vi "CSM - List Log Filter Rules As Strings.vi"(8 "Error in":errorcluster caption="Error in (no error)") -> (0 "error out":errorcluster, 2 "Rule Strings":string[](array[string]))   [LabVIEW 2020, in "Communicable State Machine.lvlib"]
uses:
  Communicable State Machine.lvlib
  LogFilter.lvclass
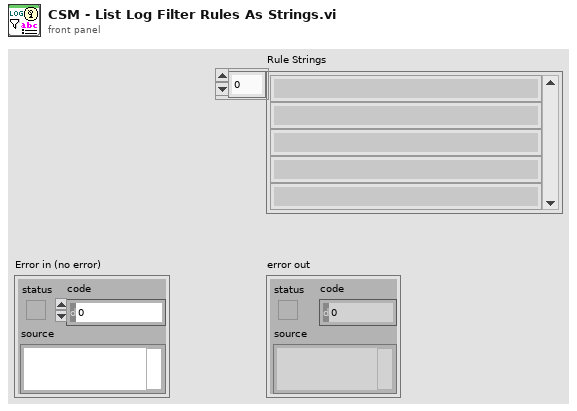
[diagram p1: front panel]
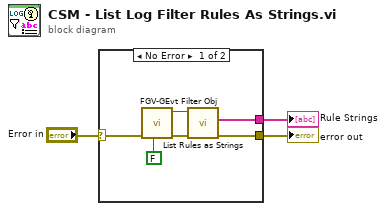
[diagram p0: block diagram]
diagram:
  n1 = case shown="No Error" "Error in" {
    selector: "Error in" -> [w6 w10]
    tunnel: [w5 w10] -> w2
    tunnel: [w4 _] -> w1
    frame No Error {
      n2 = call "FGV-GEvt Filter Obj.vi"("Set(T)/Get(F)"=FALSE, "Error in"=w6) -> ("Error out"=w8:errorcluster, "CSM:LogFilter.lvclass"=w7:refnum<class "LogFilter.lvclass">)  [unwired: 8 in]
      n3 = call "List Rules as Strings.vi"("error in (no error)"=w8, "GlobalLogFilter in"=w7) -> ("error out"=w5:errorcluster, "Rule Strings"=w4:string[])  [unwired: 7 in, 1 out]
    }
    frame Error {
    }
  }
  "error out" <- w2
  "Rule Strings" <- w1
